vi "Read String Parameter.vi"(8 "error in (no error)":errorcluster, 10 "Parameter Name":string, 11 "VoiceMeeterRemote in":refnum<class "VoiceMeeterRemote.lvclass">) -> (0 "error out":errorcluster, 2 "Value":string, 3 "VoiceMeeterRemote out":refnum<class "VoiceMeeterRemote.lvclass">)   [LabVIEW 2022 SP3, in "VoiceMeeterRemote.lvlib" / "VoiceMeeterRemote.lvclass"]
doc: "Reads a string parameter from Voicemeeter. See the VoiceMeeterRemote API manual for available parameters."
uses:
  VoiceMeeterRemote.lvclass
  VoiceMeeterRemote.lvclass/VoiceMeeterRemote.ctl
  VoiceMeeterRemote.lvlib
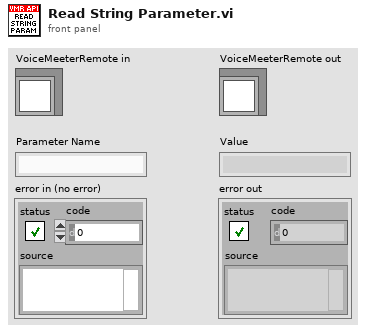
[diagram p1: front panel]
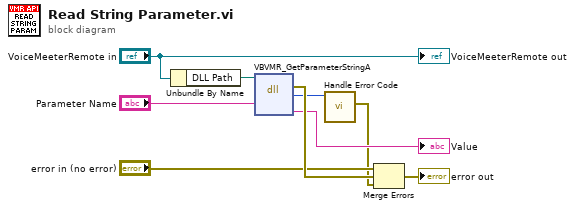
[diagram p0: block diagram]
diagram:
  n1 = Unbundle By Name("VoiceMeeterRemote in") -> ("DLL Path"=w7:path)
  n2 = dll-call lib="C:/Program Files/National Instruments/LabVIEW 2022/user.lib/VoicemeeterRemote64/VoicemeeterRemote64.*" fn="VBVMR_GetParameterStringA"(path in=w7, "szParamName"="Parameter Name") -> (error out=w9:errorcluster, "return type"=w6:i32, "szString"=→"Value":string)  [unwired: 4 in, 1 out]
  n3 = call "Handle Error Code.vi"("Code"=w6) -> ("error out"=w2:errorcluster)  [unwired: 10 in]
  n4 = Merge Errors("error in (no error)", w9, w2) -> (→"error out":errorcluster)
  "VoiceMeeterRemote out" <- "VoiceMeeterRemote in"
